vi "UnregisterTimerEvent.vi"(8 "error in (no error)":errorcluster, 10 "timer task name":string, 11 "qbus in":refnum<class "Qbus.lvclass">) -> (0 "error out":errorcluster, 3 "qbus out":refnum<class "Qbus.lvclass">)   [LabVIEW 2017, in "TimerProcess.lvlib"]
doc: "Unregisters an event with the Timer process."
uses:
  <vilib>/addons/TimerProcess/TimerProcess.lvlib
  <vilib>/addons/Qbus/Qbus.lvclass
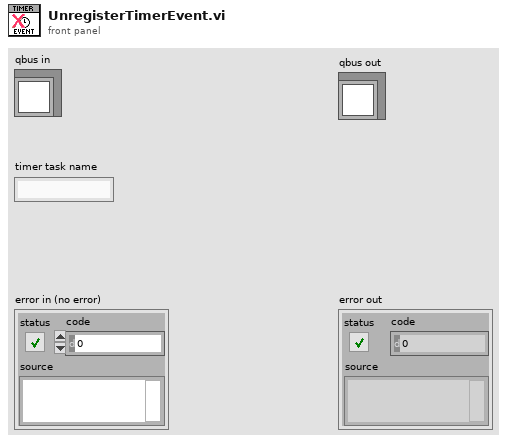
[diagram p1: front panel]
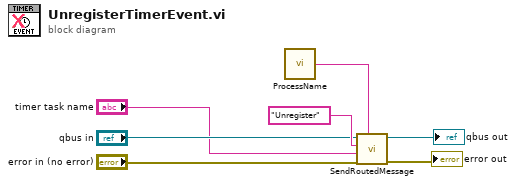
[diagram p0: block diagram]
diagram:
  n1 = call <vilib>:"ProcessName.vi"() -> ("process name"=w5:string)  [unwired: 5 in]
  n2 = call <vilib>:"SendRoutedMessage.vi"("listener process"=w5, "error in (no error)"="error in (no error)", "message value"="timer task name", "message name"="Unregister" ("MsgName"), "Qbus in"="qbus in") -> ("error in (no error)"=→"error out":errorcluster, "Qbus out"=→"qbus out":refnum<class "Qbus.lvclass">)  [unwired: 5 in]
